vi "Origin_SP (SubVI).vi"(0 "eta in":dbl[](array[numeric]), 1 "North O":dbl, 2 "East O":dbl, 5 "Set Orign":bool, 7 "eta in ship":dbl[](array[numeric]), 12 "Ring":u16(ring) items=["ROV", "Manual", "UTM"]) -> (6 "eta (local)":dbl[](array[numeric])=[-0.6740955347243753, 7.218778360091807, 28.6, 2.6878070480712677], 8 "eta ship (local)":dbl[](array[numeric]), 14 "Origin":dbl[](array[numeric]) format="%#.2f", 15 "r_n":dbl[](array[numeric]))   [LabVIEW 2014]
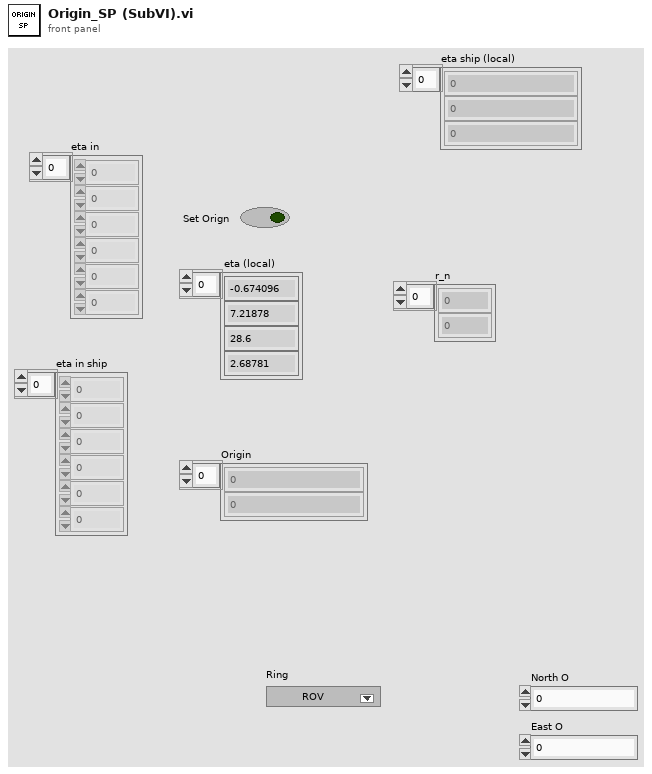
[diagram p1: front panel]
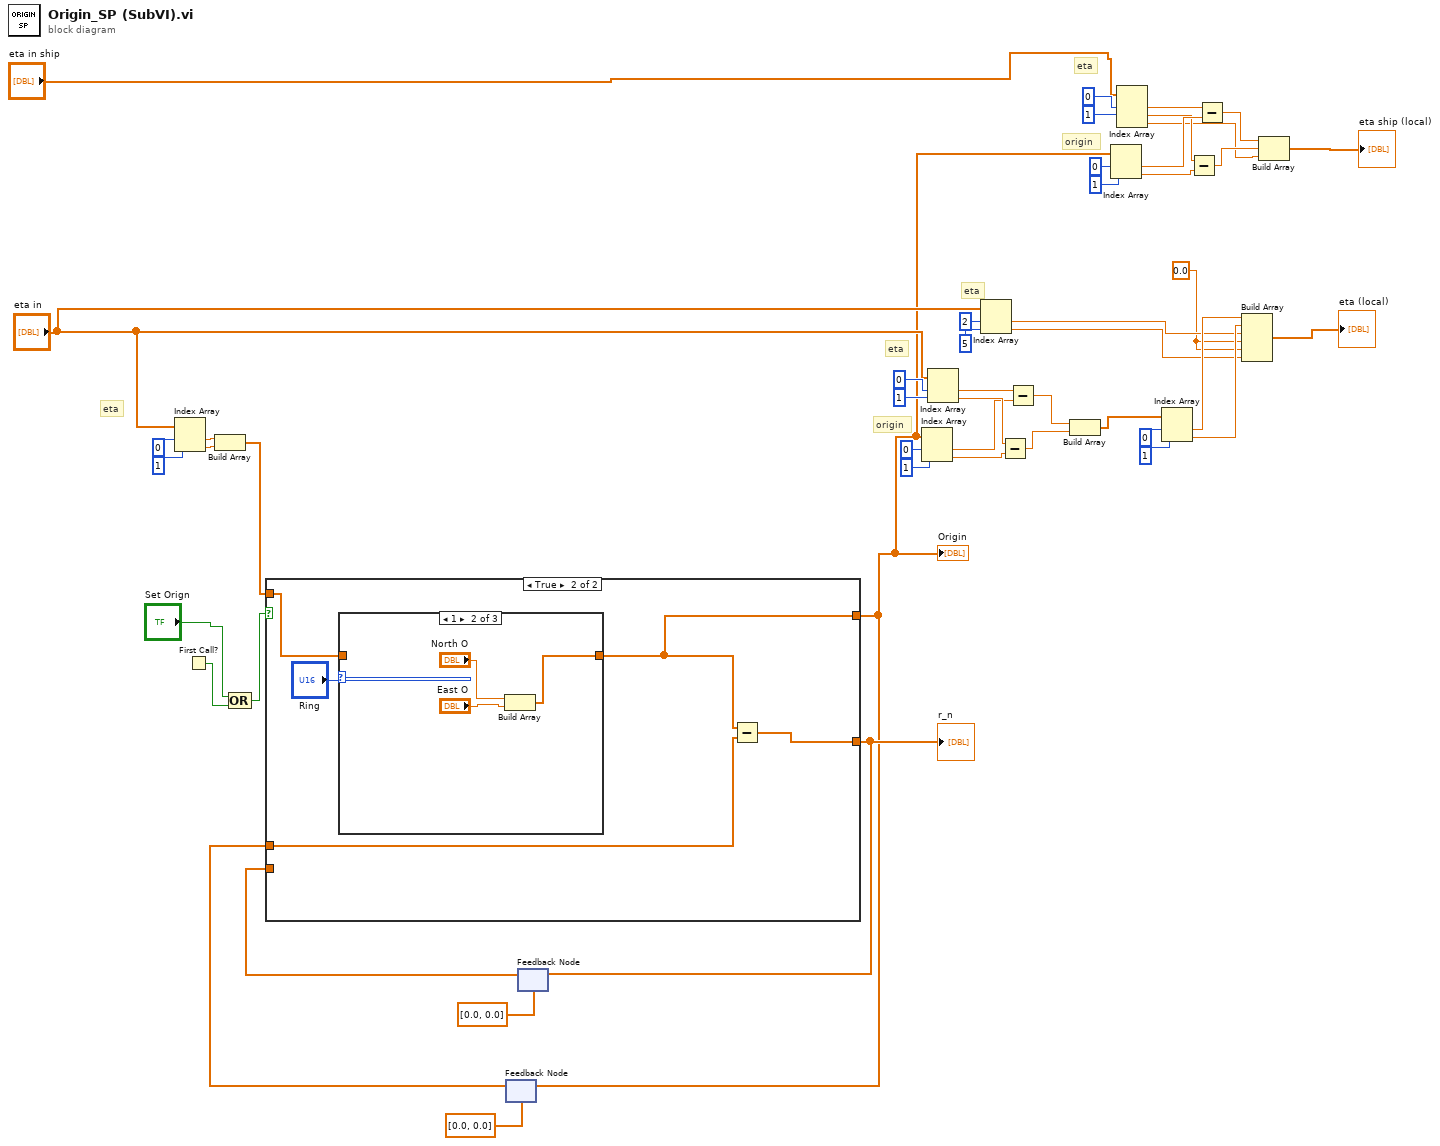
[diagram p0: block diagram]
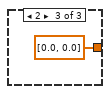
[diagram p4: hidden frame]
diagram:
  w19 = 0.0
  # "origin"
  # "eta"
  # "eta"
  # "origin"
  # "eta"
  # "eta"
  n1 = Index Array(array="eta in", index #1=0 ("index"), index #2=1 ("index")) -> (element #1=w27:dbl, element #2=w26:dbl)
  n2 = First Call?() -> (First Call?: T/F=w16:bool)
  n3 = Build Array(w27, w26) -> (w25:dbl[])
  n4 = Compound Arithmetic op=OR("Set Orign", w16) -> (w15:bool)
  n5 = feedback #1(dbl[] [0.0, 0.0]) -> (w18:dbl[])
  n6 = feedback #2(dbl[] [0.0, 0.0]) -> (w21:dbl[])
  n7 = case shown="True" w15 {
    tunnel: w25 -> [_ w55]
    tunnel: [w50 w53] -> w4
    tunnel: w18 -> [w50 w54]
    tunnel: [w51 w52] -> w22
    tunnel: w21 -> [w51 _]
    frame False {
    }
    frame True {
      n8 = case shown="1" "Ring" {
        tunnel: w55 -> [w57 _ _]
        tunnel: [w57 w58 dbl[] [0.0, 0.0]] -> w53
        frame 0, Default {
        }
        frame 1 {
          n9 = Build Array("North O", "East O") -> (w58:dbl[])
        }
        frame 2 {
        }
      }
      n10 = Subtract(x=w53, y=w54) -> (x-y=w52:dbl[])
    }
  }
  "Origin" <- w4
  "r_n" <- w22
  n11 = feedback-in #1(w4) -> ()
  n12 = feedback-in #2(w22) -> ()
  n13 = Index Array(array=w4, index #1=0 ("index"), index #2=1 ("index")) -> (element #1=w38:dbl, element #2=w40:dbl)
  n14 = Index Array(array="eta in", index #1=0 ("index"), index #2=1 ("index")) -> (element #1=w37:dbl, element #2=w39:dbl)
  n15 = Index Array(array="eta in", index #1=2 ("index"), index #2=5 ("index")) -> (element #1=w41:dbl, element #2=w20:dbl)
  n16 = Subtract(x=w39, y=w40) -> (x-y=w44:dbl)
  n17 = Subtract(x=w37, y=w38) -> (x-y=w43:dbl)
  n18 = Build Array(w43, w44) -> (w49:dbl[])
  n19 = Index Array(array=w4, index #1=0 ("index"), index #2=1 ("index")) -> (element #1=w9:dbl, element #2=w7:dbl)
  n20 = Index Array(array="eta in ship", index #1=0 ("index"), index #2=1 ("index")) -> (element #1=w10:dbl, element #2=w8:dbl, element #3=w2:dbl)  [unwired: 1 in]
  n21 = Index Array(array=w49, index #1=0 ("index"), index #2=1 ("index")) -> (element #1=w47:dbl, element #2=w48:dbl)
  n22 = Subtract(x=w8, y=w7) -> (x-y=w5:dbl)
  n23 = Subtract(x=w10, y=w9) -> (x-y=w6:dbl)
  n24 = Build Array(w47, w48, w41, w19, w19, w20) -> (→"eta (local)":dbl[])
  n25 = Build Array(w6, w5, w2) -> (→"eta ship (local)":dbl[])
